vi "DAQmx Create Channel (AI-Pressure-Bridge-Two-Point-Linear).vi"(0 "task in":refnum<k21>, 1 "maximum value":dbl=100.0 format="%0.2f", 2 "minimum value":dbl=-100.0 format="%0.2f", 3 "bridge information":T1={"bridge configuration"=10182, "voltage excitation source"=10200, "voltage excitation value"=2.5, "nominal bridge resistance"=350.0} {"voltage excitation source" items=["Internal"=10200, "External"=10167]; "bridge configuration" items=["Full Bridge"=10182, "Half Bridge"=10187, "Quarter Bridge"=10270]}, 5 "physical channels":tag, 7 "name to assign":string, 9 "units":i32(ring)=15879 items=["Pascals"=10081, "psi"=15879, "bar"=15880, "From Custom Scale"=10065], 11 "error in":errorcluster, 12 "custom scale name":tag, 14 "scaling information":T2={"first electrical value"=0.0, "second electrical value"=2.0, "electrical units"=15897, "first physical value"=0.0, "second physical value"=100.0, "physical units"=15879} {"physical units" items=["Pascals"=10081, "psi"=15879, "bar"=15880]; "electrical units" items=["Volts/Volt"=15896, "mVolts/Volt"=15897]}) -> (4 "task out":refnum<k21>, 15 "error out":errorcluster)   [LabVIEW 2024]
doc: "Creates channel(s) that use a Wheatstone bridge to measure pressure. Use this instance with sensors whose specifications do not provide a polynomial for scaling or a table of electrical and physical values. When you use this scaling type, NI-DAQmx uses two points of electrical and physical values to calculate the slope and y-intercept of a linear equation and uses that equation to scale electrical values to physical values."
uses:
  nilvaiu.dll
panel:
  # "input limits"
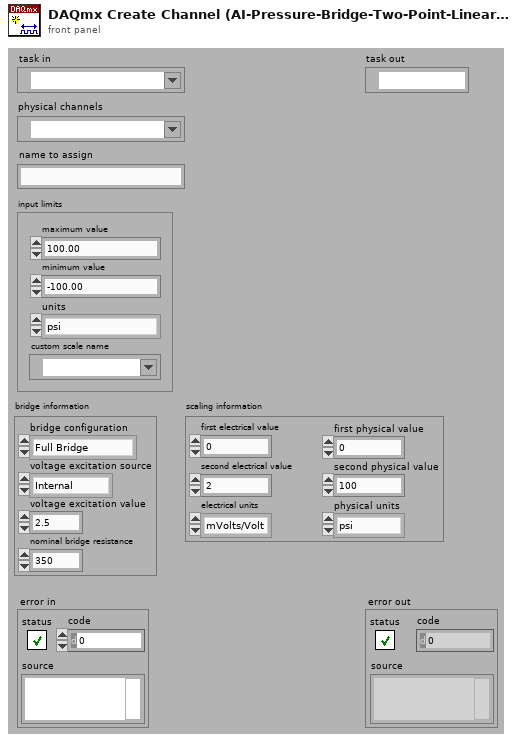
[diagram p1: front panel]
types:
  T1 = cluster{"bridge configuration":i32, "voltage excitation source":i32, "voltage excitation value":dbl, "nominal bridge resistance":dbl}
  T2 = cluster{"first electrical value":dbl, "second electrical value":dbl, "electrical units":i32, "first physical value":dbl, "second physical value":dbl, "physical units":i32}
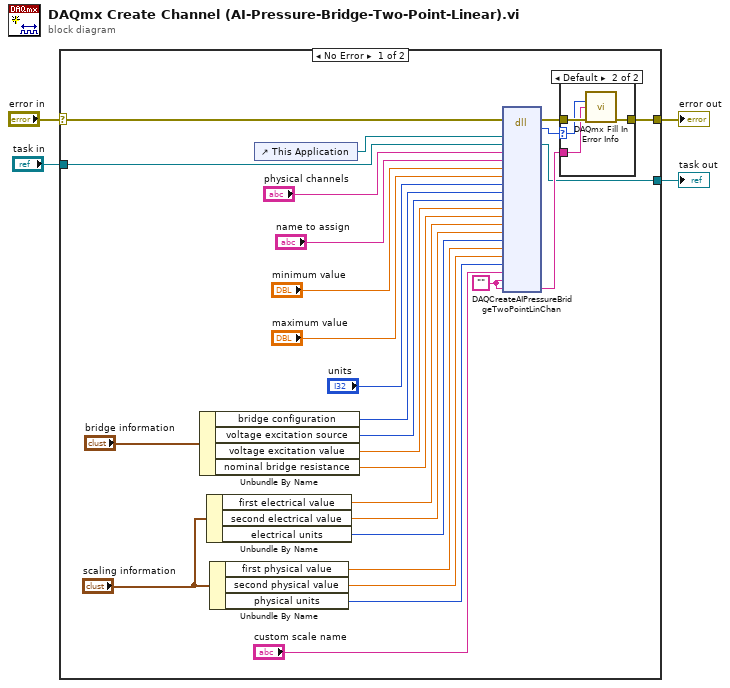
[diagram p0: block diagram]
diagram:
  n1 = case shown="No Error" "error in" {
    selector: "error in" -> [w23 w37]
    tunnel: [w26 w37] -> w4
    tunnel: "task in" -> [w8 w38]
    tunnel: [w7 w38] -> w1
    frame No Error {
      w5 = ""
      n2 = Unbundle By Name("bridge information") -> ("bridge configuration"=w13:i32, "voltage excitation source"=w12:i32, "voltage excitation value"=w11:dbl, "nominal bridge resistance"=w10:dbl)
      n3 = Unbundle By Name("scaling information") -> ("first electrical value"=w19:dbl, "second electrical value"=w18:dbl, "electrical units"=w17:i32)
      n4 = Unbundle By Name("scaling information") -> ("first physical value"=w16:dbl, "second physical value"=w15:dbl, "physical units"=w14:i32)
      n5 = control-ref of="This Application"() -> (w6:refnum<vi>)
      n6 = dll-call lib="nilvaiu.*" fn="DAQCreateAIPressureBridgeTwoPointLinChan"(error in=w23, "lvAppRef"=w6, "refObjPtr"=w8, "physicalChannelName"="physical channels", "channelNameIn"="name to assign", "minVal"="minimum value", "maxVal"="maximum value", "units"="units", "bridgeConfig"=w13, "voltageExcitSource"=w12, "voltageExcitVal"=w11, "nominalBridgeResistance"=w10, "firstElectricalValue"=w19, "secondElectricalValue"=w18, "electricalUnits"=w17, "firstPhysicalValue"=w16, "secondPhysicalValue"=w15, "physicalUnits"=w14, "customScaleName"="custom scale name", "channelNamesOut"=w5, "extendedErrorInfo"=w5) -> (error out=w29:errorcluster, "return type"=w28:i32, "refObjPtr"=w7:refnum<k21>, "extendedErrorInfo"=w27:string)  [unwired: 20 in, 1 out]
      n7 = case shown="Default" w28 {
        selector: w28 -> [_ w34]
        tunnel: w29 -> [w32 w36]
        tunnel: [w32 w35] -> w26
        tunnel: w27 -> [_ w33]
        frame 0 {
        }
        frame Default {
          n8 = call "DAQmx Fill In Error Info.vi"("status code"=w34, "extended error info"=w33, "error in"=w36) -> ("error out"=w35:errorcluster)  [unwired: 1 in, 11 out]
        }
      }
    }
    frame Error {
    }
  }
  "error out" <- w4
  "task out" <- w1
